vi "tm3samp_sequence.vi"() -> ()   [LabVIEW 2011]
panel:
  out "Image":u16[][](graph)
  out "Frames Per Second":dbl
  in  "Quit":bool
  out "Error Out":errorcluster
  # "This is just a simple example of how to create a sequence\ncapture from start to finish."
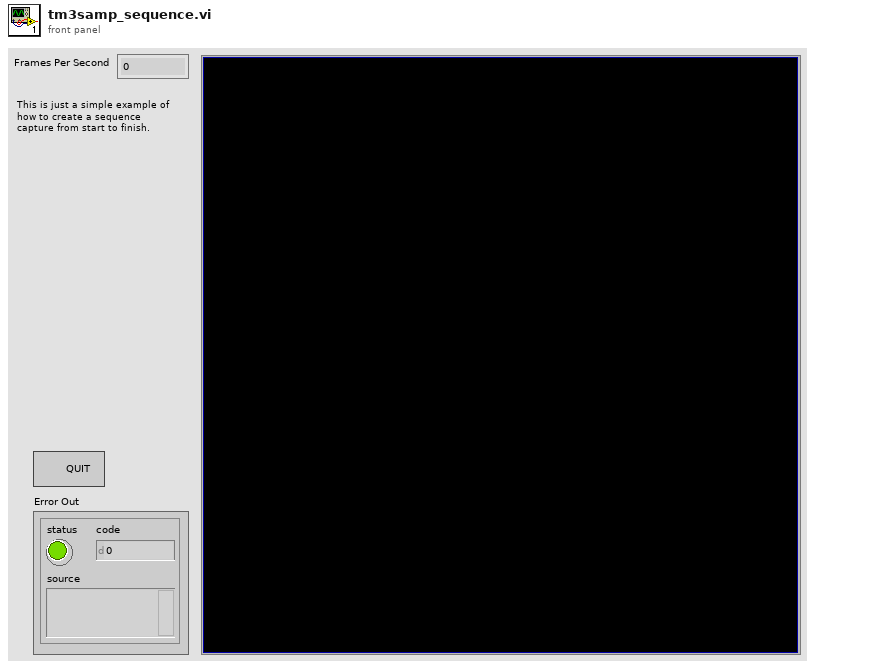
[diagram p1: front panel]
types:
  T1 = cluster{"width":u32, "height":u32, "datatype":u32}
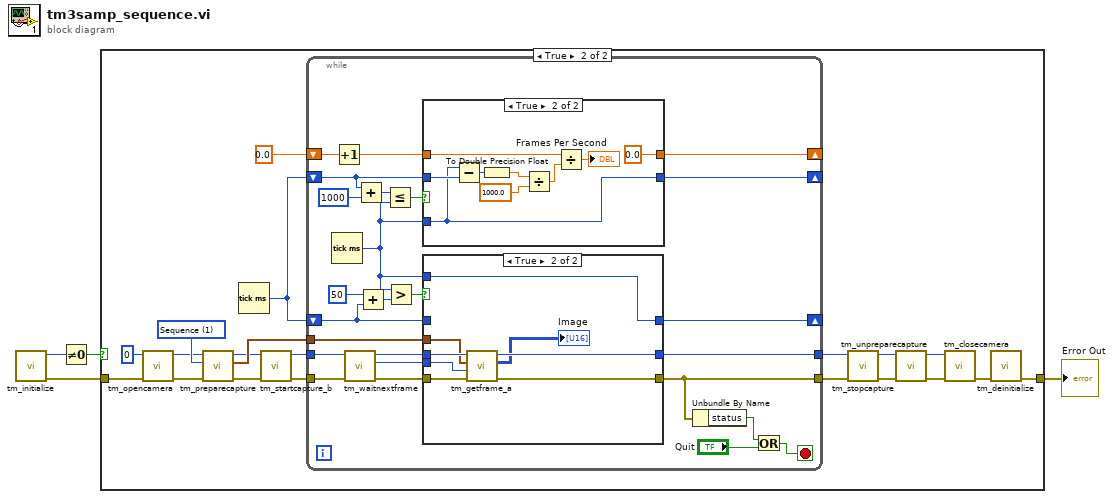
[diagram p0: block diagram]
diagram:
  n1 = call <userlib>:"tm_initialize.vi"() -> ("error out"=w1:errorcluster, "Number Of Cameras"=w2:u32)  [unwired: 10 in]
  n2 = Not Equal To 0?(x=w2) -> (x != 0?=w4:bool)
  n3 = case shown="True" w4 {
    tunnel: w1 -> [w5 w25]
    tunnel: [w5 w22] -> w3
    frame False {
    }
    frame True {
      w13 = 1 items=["Snap", "Sequence"] ("Capture mode")
      n4 = call <userlib>:"tm_opencamera.vi"("error in (no error)"=w25, "Camera Index"=u32 0) -> ("error out"=w7:errorcluster, "Handle out"=w8:u32)  [unwired: 8 in]
      n5 = call <userlib>:"tm_preparecapture.vi"("error in (no error)"=w7, "Capture mode"=w13, "Handle in"=w8) -> ("error out"=w10:errorcluster, "Buffer"=w12:T1, "Handle out"=w11:u32)  [unwired: 5 in, 1 out]
      n6 = Tick Count (ms)() -> (millisecond timer value=w6:u32)
      n7 = call <userlib>:"tm_startcapture_b.vi"("error in (no error)"=w10, "Handle in"=w11) -> ("error out"=w14:errorcluster, "Handle out"=w15:u32)  [unwired: 8 in]
      n8 = while {
        tunnel: [w29] -> w18
        tunnel: [w30] -> w19
        tunnel: w12 -> [w27]
        tunnel: w15 -> [w47]
        tunnel: w14 -> [w48]
        shift-right: [w45] -> _
        shift-left: w6 -> [w42]
        shift-right: [w46] -> _
        shift-left: 0.0 -> [w39]
        shift-right: [w28] -> _
        shift-left: w6 -> [w31]
        stop <- w26 stop-if-true
        n9 = Tick Count (ms)() -> (millisecond timer value=w32:u32)
        n10 = Increment(x=w39) -> (x+1=w40:dbl)
        n11 = call <userlib>:"tm_waitnextframe.vi"("error in (no error)"=w48, "Handle in"=w47) -> ("error out"=w37:errorcluster, "Frame Index"=w36:i32, "Handle out"=w38:u32)  [unwired: 6 in, 1 out]
        n12 = Add(x=w42, y=u32 1000) -> (x+y=w44:u32)
        n13 = Add(x=u32 50, y=w31) -> (x+y=w34:u32)
        n14 = Less Or Equal?(x=w44, y=w32) -> (x <= y?=w41:bool)
        n15 = Greater?(x=w32, y=w34) -> (0:w33:bool)
        n16 = case shown="True" w41 {
          tunnel: w42 -> [w63 w66]
          tunnel: [w63 w64] -> w45
          tunnel: w40 -> [w62 w70]
          tunnel: w32 -> [_ w64]
          tunnel: [w62 0.0] -> w46
          frame False {
          }
          frame True {
            n17 = Subtract(x=w64, y=w66) -> (x-y=w65:u32)
            n18 = To Double Precision Float(number=w65) -> (double precision float=w72:dbl)
            n19 = Divide(x=w72, y=1000.0) -> (x/y=w69:dbl)
            n20 = Divide(x=w70, y=w69) -> (x/y=→"Frames Per Second":dbl)
          }
        }
        n21 = case shown="True" w33 {
          tunnel: w38 -> [w53 w61]
          tunnel: w37 -> [w52 w60]
          tunnel: w36 -> [_ w59]
          tunnel: w31 -> [w51 _]
          tunnel: w32 -> [_ w58]
          tunnel: [w53 w55] -> w29
          tunnel: [w52 w56] -> w30
          tunnel: [w51 w58] -> w28
          tunnel: w27 -> [_ w57]
          frame False {
          }
          frame True {
            n22 = call <userlib>:"tm_getframe_a.vi"("error in (no error)"=w60, "Frame Index"=w59, "Buffer"=w57, "Handle in"=w61) -> ("error out"=w56:errorcluster, "Data 16"=→"Image":u16[][], "Handle out"=w55:u32)  [unwired: 3 in, 2 out]
          }
        }
        n23 = Unbundle By Name(w30) -> ("status"=w50:bool)
        n24 = Or(x=w50, y="Quit") -> (x .or. y?=w26:bool)
      }
      n25 = call <userlib>:"tm_stopcapture.vi"("error in (no error)"=w19, "Handle in"=w18) -> ("error out"=w16:errorcluster, "Handle out"=w17:u32)  [unwired: 8 in]
      n26 = call <userlib>:"tm_unpreparecapture.vi"("error in (no error)"=w16, "Handle in"=w17) -> ("error out"=w21:errorcluster, "Handle out"=w20:u32)  [unwired: 8 in]
      n27 = call <userlib>:"tm_closecamera.vi"("error in (no error)"=w21, "Handle in"=w20) -> ("error out"=w23:errorcluster)  [unwired: 9 in]
      n28 = call <userlib>:"tm_deinitialize.vi"("error in (no error)"=w23) -> ("error out"=w22:errorcluster)  [unwired: 10 in]
    }
  }
  "Error Out" <- w3
